vi "Release.vi"(0 "Execution in":refnum<class "Execution.lvclass">, 11 "error in (no error)":errorcluster) -> (4 "Execution out":refnum<class "Execution.lvclass">, 15 "error out":errorcluster)   [LabVIEW 2020]
uses:
  VariableContainer/VariableContainer.lvclass
  SequenceFile/SequenceFile.lvclass
  SequenceFile/Typedefs/Session Handle.ctl
  VariableContainer/Typedefs/Session Handle.ctl
  Execution.lvclass
  C:/Program Files (x86)/National Instruments/LabVIEW 2020/user.lib/_Session Fwk/Session - Root.lvclass
  C:/dev/HTS/Execution/Execution.lvclass
  C:/dev/HTS/SequenceFile/SequenceFile.lvclass
  C:/dev/HTS/VariableContainer/VariableContainer.lvclass
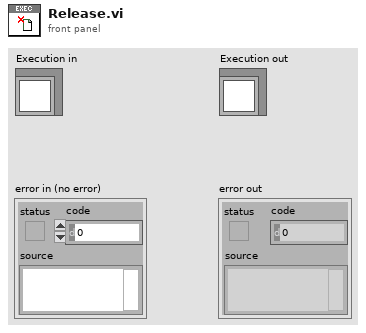
[diagram p1: front panel]
types:
  T1 = typedef "HTS.lvlib/VariableContainer.lvclass/Session Handle.ctl" = refnum<data-value>
  T2 = typedef "HTS.lvlib/SequenceFile.lvclass/Session Handle.ctl" = refnum<data-value>
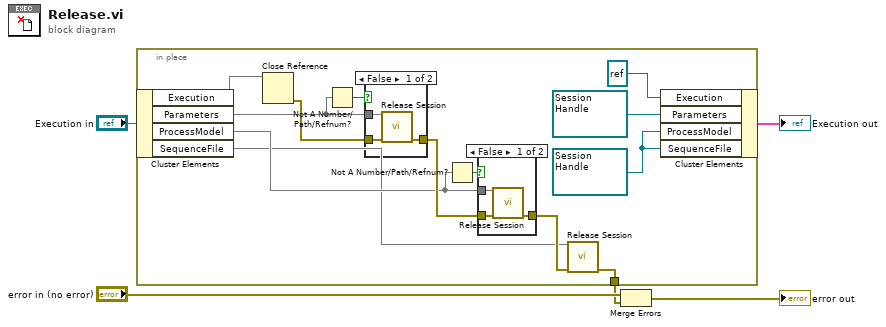
[diagram p0: block diagram]
diagram:
  n1 = in-place {
    in-place-border: [w6] -> w1
    w9 = T2 refnum ("SequenceFile")
    n2 = in-place-cluster #1("Execution in") -> ("Execution"=w12, "Parameters"=w13, "ProcessModel"=w11, "SequenceFile"=w10)
    n3 = Close Reference(reference=w12) -> (error out=w18:errorcluster)  [unwired: 1 in]
    n4 = Not A Number/Path/Refnum?(number/path/refnum=w13) -> (NaN/Path/Refnum?=w15:bool)
    n5 = case shown="False" w15 {
      tunnel: w18 -> [w25 w26]
      tunnel: [w24 w26] -> w17
      tunnel: w13 -> [w23 _]
      frame False {
        n6 = call "Release Session.vi"("Session Handle"=w23, "error in (no error)"=w25) -> ("error out"=w24:errorcluster)  [unwired: 13 in]
      }
      frame True {
      }
    }
    n7 = Not A Number/Path/Refnum?(number/path/refnum=w11) -> (NaN/Path/Refnum?=w14:bool)
    n8 = case shown="False" w14 {
      tunnel: w11 -> [w21 _]
      tunnel: w17 -> [w20 w22]
      tunnel: [w19 w22] -> w16
      frame False {
        n9 = call "Release Session.vi"("Session Handle"=w21, "error in (no error)"=w20) -> ("error out"=w19:errorcluster)  [unwired: 13 in]
      }
      frame True {
      }
    }
    n10 = call "Release Session.vi"("Session Handle"=w10, "error in (no error)"=w16) -> ("error out"=w6:errorcluster)  [unwired: 13 in]
    n11 = in-place-cluster #1("Execution"=refnum<k7> refnum, "Parameters"=T1 refnum, "ProcessModel"=w9, "SequenceFile"=w9) -> (→"Execution out":cluster{})
  }
  n12 = Merge Errors("error in (no error)", w1) -> (→"error out":errorcluster)
